vi "read_nsalex_photon_hdf5.vi"() -> ()   [LabVIEW 2010]
uses:
  <vilib>/addons/h5labview2/file/H5F.lvlib
  <vilib>/addons/h5labview2/file/H5Fmode.ctl
  <vilib>/addons/h5labview2/group/H5G.lvlib
  <vilib>/addons/h5labview2/dataset/H5Dread.llb/H5Dread.xnode
  <vilib>/addons/h5labview2/base/H5Equery.vi
  <vilib>/addons/h5labview2/base/lib_path.vi
  <vilib>/Analysis/NI_AALBase.lvlib
  <vilib>/addons/h5labview2/base/hid_t.ctl
  <vilib>/Analysis/1siggen.llb/Ramp Pattern by Delta.vi
panel:
  out "tcspc_range":dbl
  out "tcspc_num_bins":i32
  out "laser_repetion_rate":u32
  out "measurement_type":string
  out "tcspc_unit":dbl
  out "nanotimes":u16[](array[numeric])
  out "error out":errorcluster
  out "Nanotime Histograms":cluster{"Ramp Pattern":dbl[], u32[]}[](graph)
  out "acceptor_period":u32[](array[numeric])
  out "donor_period":u32[](array[numeric])
  out "spectral_ch2":u32[](array[numeric])
  out "spectral_ch1":u32[](array[numeric])
  out "detectors":u32[](array[numeric])
  out "timestamps_unit":dbl
  out "timestamps":i64[](array[numeric])
  in  "Path":path
  # "(C) 2015 the Regents of the University of California\n\nAuthors: X. Michalet (UCLA)"
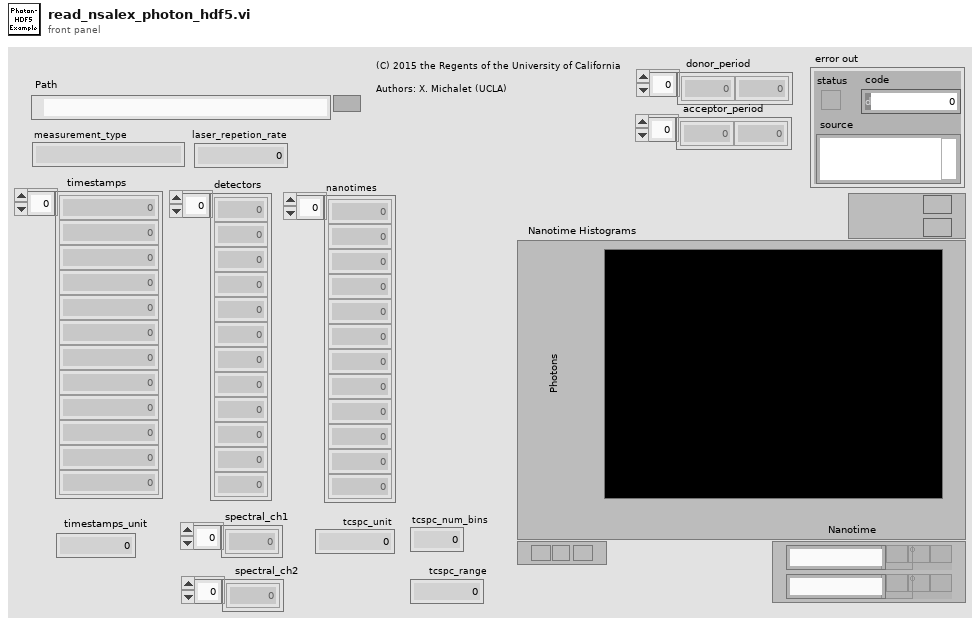
[diagram p1: front panel]
types:
  T1 = typedef "H5F.lvlib/H5Fmode.ctl" = enum16{"read-only", "read-write", "overwrite", "create new", "open or create"}
  T2 = typedef "hid_t.ctl" = i32
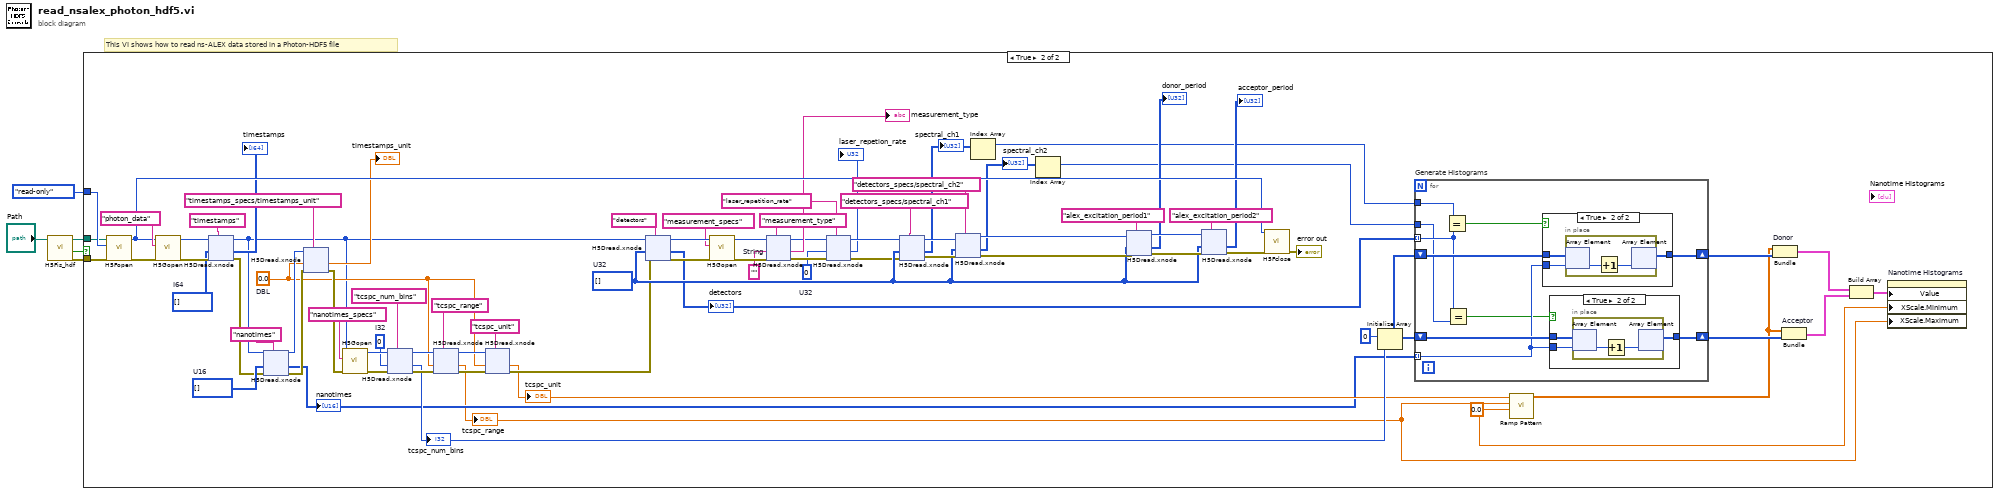
[diagram p0: block diagram]
diagram:
  # "This VI shows how to read ns-ALEX data stored in a Photon-HDF5 file"
  n1 = call <vilib>:"H5Fis_hdf.vi"("path in"="Path") -> ("error out"=w1:errorcluster, "valid?"=w2:bool, "path out"=w3:path)  [unwired: 7 in, 1 out]
  n2 = case shown="True" w2 {
    tunnel: H5Fmode."read-only" ("mode (read-only)") -> [_ w87]
    tunnel: w3 -> [_ w86]
    tunnel: w1 -> [_ w85]
    frame False {
    }
    frame True {
      w20 = 0  # I32
      w33 = u32 0  # U32
      w44 = ""  # String
      w52 = u16[] []  # U16
      w7 = 0.0 ("start")
      w60 = u32[] []  # U32
      w18 = 0.0  # DBL
      w79 = i64[] []  # I64
      n3 = call <vilib>:"H5Fopen.vi"("error in (no error)"=w85, "mode (read-only)"=w87, "path"=w86) -> ("error out"=w84:errorcluster, "ref out"=w57:T2)  [unwired: 7 in]
      n4 = call <vilib>:"H5Gopen.vi"("error in (no error)"=w84, "name"="photon_data", "ref in"=w57) -> ("error out"=w80:errorcluster, "group out"=w82:T2)  [unwired: 7 in]
      n5 = xnode "H5Dread.xnode"("dataset name (this)"="timestamps", "error in (no error)"=w80, "default"=w79, "ref in"=w82) -> ("error out"=w49:errorcluster, "data"=→"timestamps":i64[], "ref out"=w8:i32)  [unwired: 2 in, 1 out]
      n6 = xnode "H5Dread.xnode"("dataset name (this)"="nanotimes", "error in (no error)"=w49, "default"=w52, "ref in"=w8) -> ("error out"=w48:errorcluster, "data"=w15:u16[], "ref out"=w51:i32)  [unwired: 2 in, 1 out]
      "nanotimes" <- w15
      n7 = xnode "H5Dread.xnode"("dataset name (this)"="timestamps_specs/timestamps_unit" ("object name"), "error in (no error)"=w48, "default"=w18, "ref in"=w51) -> ("error out"=w42:errorcluster, "data"=→"timestamps_unit":dbl)  [unwired: 2 in, 2 out]
      n8 = call <vilib>:"H5Gopen.vi"("error in (no error)"=w42, "name"="nanotimes_specs" ("object name"), "ref in"=w8) -> ("error out"=w24:errorcluster, "group out"=w27:T2)  [unwired: 7 in]
      n9 = xnode "H5Dread.xnode"("dataset name (this)"="tcspc_num_bins" ("object name"), "error in (no error)"=w24, "default"=w20, "ref in"=w27) -> ("error out"=w23:errorcluster, "data"=w17:i32, "ref out"=w26:i32)  [unwired: 2 in, 1 out]
      "tcspc_num_bins" <- w17
      n10 = xnode "H5Dread.xnode"("dataset name (this)"="tcspc_range" ("object name"), "error in (no error)"=w23, "default"=w18, "ref in"=w26) -> ("error out"=w22:errorcluster, "data"=w6:dbl, "ref out"=w25:i32)  [unwired: 2 in, 1 out]
      "tcspc_range" <- w6
      n11 = xnode "H5Dread.xnode"("dataset name (this)"="tcspc_unit" ("object name"), "error in (no error)"=w22, "default"=w18, "ref in"=w25) -> ("error out"=w39:errorcluster, "data"=w16:dbl)  [unwired: 2 in, 2 out]
      "tcspc_unit" <- w16
      n12 = xnode "H5Dread.xnode"("dataset name (this)"="detectors", "error in (no error)"=w39, "default"=w60, "ref in"=w8) -> ("error out"=w74:errorcluster, "data"=w12:u32[], "ref out"=w76:i32)  [unwired: 2 in, 1 out]
      "detectors" <- w12
      n13 = call <vilib>:"H5Gopen.vi"("error in (no error)"=w74, "name"="measurement_specs" ("object name"), "ref in"=w76) -> ("error out"=w47:errorcluster, "group out"=w46:T2)  [unwired: 7 in]
      n14 = xnode "H5Dread.xnode"("dataset name (this)"="measurement_type" ("object name"), "error in (no error)"=w47, "default"=w44, "ref in"=w46) -> ("error out"=w38:errorcluster, "data"=→"measurement_type":string, "ref out"=w36:i32)  [unwired: 2 in, 1 out]
      n15 = xnode "H5Dread.xnode"("dataset name (this)"="laser_repetition_rate" ("object name"), "error in (no error)"=w38, "default"=w33, "ref in"=w36) -> ("error out"=w37:errorcluster, "data"=→"laser_repetion_rate":u32, "ref out"=w35:i32)  [unwired: 2 in, 1 out]
      n16 = xnode "H5Dread.xnode"("dataset name (this)"="detectors_specs/spectral_ch1", "error in (no error)"=w37, "default"=w60, "ref in"=w35) -> ("error out"=w72:errorcluster, "data"=w14:u32[], "ref out"=w71:i32)  [unwired: 2 in, 1 out]
      "spectral_ch1" <- w14
      n17 = xnode "H5Dread.xnode"("dataset name (this)"="detectors_specs/spectral_ch2", "error in (no error)"=w72, "default"=w60, "ref in"=w71) -> ("error out"=w68:errorcluster, "data"=w13:u32[], "ref out"=w69:T2)  [unwired: 2 in, 1 out]
      "spectral_ch2" <- w13
      n18 = Index Array(array=w14) -> (element=w11:u32)  [unwired: 1 in]
      n19 = Index Array(array=w13) -> (element=w10:u32)  [unwired: 1 in]
      n20 = xnode "H5Dread.xnode"("dataset name (this)"="alex_excitation_period1", "error in (no error)"=w68, "default"=w60, "ref in"=w69) -> ("error out"=w65:errorcluster, "data"=→"donor_period":u32[], "ref out"=w66:i32)  [unwired: 2 in, 1 out]
      n21 = xnode "H5Dread.xnode"("dataset name (this)"="alex_excitation_period2", "error in (no error)"=w65, "default"=w60, "ref in"=w66) -> ("error out"=w59:errorcluster, "data"=→"acceptor_period":u32[])  [unwired: 2 in, 2 out]
      n22 = call <vilib>:"H5Fclose.vi"("error in (no error)"=w59, "ref"=w57) -> ("error out"=→"error out":errorcluster)  [unwired: 9 in]
      n23 = Initialize Array(u32 0 ("element"), w17) -> (w54:u32[])
      n24 = for "Generate Histograms" {
        shift-right: [w187] -> w62
        shift-left: w54 -> [w186]
        shift-right: [w184] -> w61
        shift-left: w54 -> [w185]
        tunnel: w15 -> [w183] mode=indexing
        tunnel: w12 -> [w180] mode=indexing
        tunnel: w11 -> [w182]
        tunnel: w10 -> [w178]
        n25 = Equal?(x=w182, y=w180) -> (x = y?=w181:bool)
        n26 = Equal?(x=w180, y=w178) -> (x = y?=w179:bool)
        n27 = case shown="True" w181 {
          tunnel: [w194 w196] -> w187
          tunnel: w186 -> [w194 w197]
          tunnel: w183 -> [_ w195]
          frame False {
          }
          frame True {
            n28 = in-place {
              n29 = in-place-array #1(w197, w195) -> (w199:u32)
              n30 = Increment(x=w199) -> (x+1=w198:u32)
              n31 = in-place-array #1(w198) -> (w196:u32[])  [unwired: 1 out]
            }
          }
        }
        n32 = case shown="True" w179 {
          tunnel: [w188 w190] -> w184
          tunnel: w185 -> [w188 w191]
          tunnel: w183 -> [_ w189]
          frame False {
          }
          frame True {
            n33 = in-place {
              n34 = in-place-array #2(w191, w189) -> (w193:u32)
              n35 = Increment(x=w193) -> (x+1=w192:u32)
              n36 = in-place-array #2(w192) -> (w190:u32[])  [unwired: 1 out]
            }
          }
        }
      }
      n37 = call-poly <vilib>:"Ramp Pattern.vi"("start"=w7, "end"=w6, "delta"=w16) -> ("Ramp Pattern"=w55:dbl[])  [unwired: 6 in, 2 out]
      n38 = Bundle "Donor"("Ramp Pattern"=w55, w62) -> (w30:cluster{"Ramp Pattern":dbl[], u32[]})  [unwired: 1 in]
      n39 = Bundle "Acceptor"("Ramp Pattern"=w55, w61) -> (w29:cluster{"Ramp Pattern":dbl[], u32[]})  [unwired: 1 in]
      n40 = Build Array(w30, w29) -> (w9:cluster{"Ramp Pattern":dbl[], u32[]}[])
      n41 = property on="Nanotime Histograms" class="XYGraph (strict)"("Value"=w9, "XScale.Minimum"=w7, "XScale.Maximum"=w6) -> ()  [unwired: 2 in, 2 out]
    }
  }
